vi "运维调试_氨氮.vi"() -> ()   [LabVIEW 2016, in "斯坦道氨氮.lvlib"]
uses:
  <vilib>/Utility/miscctls.llb/LVPointTypeDef.ctl
  <vilib>/Utility/config.llb/NI_LVConfig.lvlib
  <vilib>/ptbypt/NI_PtbyPt.lvlib
panel:
  in  "仪器参数设置":bool
  in  "模块启用":bool
  in  "串口设置":bool
  in  "备用系数一键写入":bool
  in  "公式一键写入":bool
  in  "流程路径":path=path "C:/Users/STD/Documents/斯坦道流程文件/流程.xml"
  in  "曲线模型":cluster{"X^2":dbl, "X":dbl, "B":dbl}(xcontrol)
  out "字符串":string
  in  "质控参数设置":bool
  in  "自动测试量程配置":T1
  out "温度2":sgl
  out "温度1":sgl
  out "ADC":sgl
  out "固件版本号":string
  in  "数组":string[](array[string])
  in  "备用系数写入":bool
  in  "备用系数读取":bool
  in  "备用系数":T2
  in  "量程切换阈值写入":bool
  in  "量程切换阈值读取":bool
  in  "量程切换阈值":cluster{"阈值":dbl, "标液浓度":dbl}
  in  "参数下拉列表":enum16{"总磷", "总氮", "氨氮"}(ring)=enum."氨氮"
  in  "量程下拉列表":enum16{"低量程", "高量程"}(ring)
  in  "测量模式下拉列表":enum16{"水样测量", "零点核查", "跨度核查", "标样核查", "加标回收"}(ring)
  in  "公式":cluster{"X^2":dbl, "X":dbl, "b":dbl}
  in  "写公式":bool
  in  "读公式":bool
  in  "返回":bool
  in  "设置":bool
  out "序列号":string="序列号"
  out "测量数据":T3(xcontrol)
  out "集成报警信息":string
  out "定时启动":bool
  out "运行状态":T4(xcontrol)
  in  "停止":bool
  in  "手动启动":bool
  in  "单步测试":bool
  in  "总磷氨氮调试":u16[](xcontrol)
  out "F3":sgl format="%#.6f"
  out "F2":sgl format="%#.6f"
  out "F1":sgl format="%#.6f"
  out "F0":sgl format="%#.6f"
  out "多列列表框":i32(listbox)
  # "参数设置"
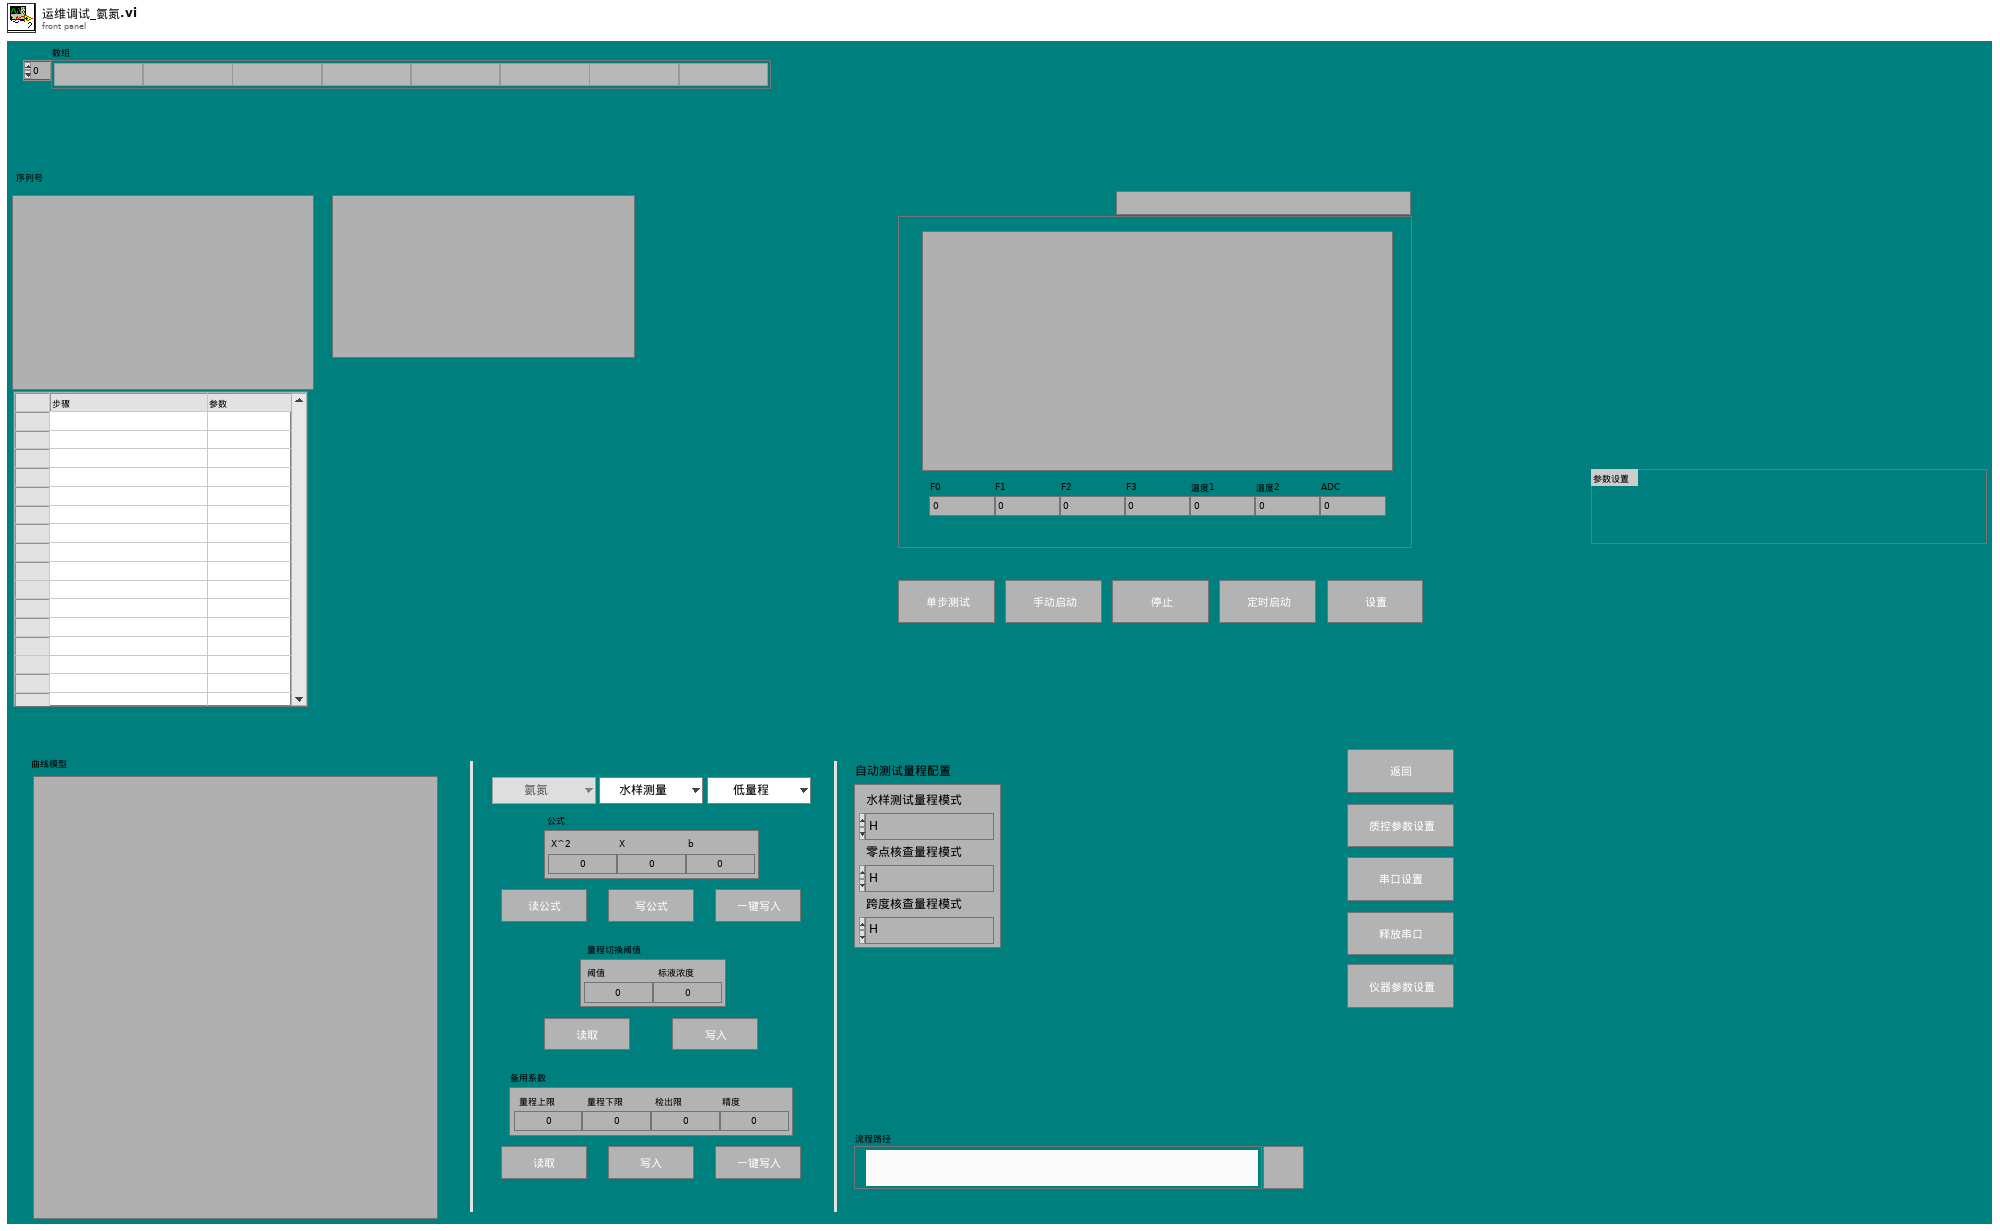
[diagram p1: front panel]
types:
  T1 = cluster{"水样测试量程模式":enum16{"H", "L", "AUTO"}, "空白核查量程模式":enum16{"H", "L", "AUTO"}, "跨度核查量程模式":enum16{"H", "L", "AUTO"}}
  T2 = cluster{"量程上限":dbl, "量程下限":dbl, "检出限":dbl, "精度":dbl}
  T3 = cluster{"flowid":u16, "测量精度":u16, "测量数据区":cluster{"因子编码":u32, "单位":u16, "标样参考值":sgl, "水样数据时间":timestamp, "水样实测值":sgl, "水样数据标识":string, "标样数据时间":timestamp, "标样实测值":sgl, "标样数据标识":string, "空白数据时间":timestamp, "空白实测值":sgl, "空白数据标识":string, "零点核查数据时间":timestamp, "零点核查实测值":sgl, "零点核查数据标识":string, "跨度核查数据时间":timestamp, "跨度核查实测值":sgl, "跨度核查数据标识":string, "加标回收数据时间":timestamp, "加标回收实测值":sgl, "加标回收数据标识":string, "平行样数据时间":timestamp, "平行样实测值":sgl, "平行样数据标识":string, "F0":sgl, "F1":sgl, "F2":sgl, "F3":sgl, "F4":sgl, "F5":sgl, "F6":sgl, "F7":sgl, "温度":sgl, "湿度":sgl, "X值":sgl}}
  T4 = cluster{"系统时间":timestamp, "工作状态":enum16{"空闲", "水样测试", "标样核查", "零点核查", "跨度核查", "空白测试", "平行样测试", "加标回收", "空白校准", "标样校准", "初始化（清洗）"}, "测量模式":enum16{"待机", "连续模式", "周期模式", "定点模式", "受控模式", "手动模式"}, "告警代码":enum16{"无告警", "缺试剂告警", "缺水样告警", "缺蒸馏水告警", "缺标液告警", "仪表漏液告警", "标定异常告警", "超量程告警", "加热异常", "低试剂预警", "超上限告警", "超下限告警", "仪表内部其他异常", "滴定异常告警", "电极异常告警", "量程切换告警", "参数设置告警", "PH电极电位异常", "电导率电极异常", "浊度光度异常", "溶解氧电极异常", "溶解氧光强异常", "温度异常告警", "PH异常告警", "溶解氧异常告警", "电导率异常告警", "浊度异常告警", "叶绿素异常告警", "藻密度异常告警", "蓝绿藻异常告警", "ORP异常告警", "氨氮异常告警", "清洁刷异常告警", "SD卡异常告警", "蓝牙异常告警", "Wifi异常告警", "流程异常告警"}, "故障代码":enum16{"无故障", "电机故障", "温度故障", "通讯故障", "滴定故障"}, "日志代码":u16, "软件版本":u16, "F0":sgl, "F1":sgl, "F2":sgl, "F3":sgl, "T":sgl, "H":sgl, "id":u16, "flowid":u16, "量程":u16, "总磷控温温度1":sgl, "营养盐控温温度2":sgl, "ADC":sgl}
  T5 = enum16{"启动测量", "标样核查", "零点核查", "跨度核查", "空白测试", "平行样测试", "加标回收", "空白校准", "标样校准", "初始化（清洗）", "停止测试", "仪器重启", "校时", "模式设置", "测量间隔设置"}
  T6 = cluster{"控制命令":enum16{"启动测量", "标样核查", "零点核查", "跨度核查", "空白测试", "平行样测试", "加标回收", "空白校准", "标样校准", "初始化（清洗）", "停止测试", "仪器重启", "校时", "模式设置", "测量间隔设置"}, "周期设置类型":enum16{"定点启动", "间隔启动"}, "定时功能启用":bool, "定时间隔":dbl, "24H周期设置":bool[], "零点核查时间":u16, "跨度核查时间":u16, "质控频次":enum16{"关闭", "每天", "星期一", "星期二", "星期三", "星期四", "星期五", "星期六", "星期日"}}
  T7 = enum16{"关闭", "每天", "星期一", "星期二", "星期三", "星期四", "星期五", "星期六", "星期日"}
  T8 = typedef "LVDateTimeRec.ctl" = cluster{"秒数的小数部分":dbl, "秒":i32, "分":i32, "时":i32, "日":i32, "月":i32, "年":i32, "天数（周）":i32, "天数（年）":i32, "DST":i32}
  T9 = enum16{"空闲", "水样测试", "标样核查", "零点核查", "跨度核查", "空白测试", "平行样测试", "加标回收", "空白校准", "标样校准", "初始化（清洗）"}
  T10 = enum32{"Bad", "Idle", "Run top level", "Running"}
  T11 = typedef "LVPointTypeDef.ctl" = cluster{"Horizontal":i16, "Vertical":i16}
  T12 = cluster{"因子编码":u32, "单位":u16, "标样参考值":sgl, "水样数据时间":timestamp, "水样实测值":sgl, "水样数据标识":string, "标样数据时间":timestamp, "标样实测值":sgl, "标样数据标识":string, "空白数据时间":timestamp, "空白实测值":sgl, "空白数据标识":string, "零点核查数据时间":timestamp, "零点核查实测值":sgl, "零点核查数据标识":string, "跨度核查数据时间":timestamp, "跨度核查实测值":sgl, "跨度核查数据标识":string, "加标回收数据时间":timestamp, "加标回收实测值":sgl, "加标回收数据标识":string, "平行样数据时间":timestamp, "平行样实测值":sgl, "平行样数据标识":string, "F0":sgl, "F1":sgl, "F2":sgl, "F3":sgl, "F4":sgl, "F5":sgl, "F6":sgl, "F7":sgl, "温度":sgl, "湿度":sgl, "X值":sgl}
  T13 = typedef "NI_LVConfig.lvlib/Config Data RefNum.ctl" = refnum<k1>
  T14 = cluster{"参数下拉列表":enum16{"总磷", "总氮", "氨氮"}, "测量模式下拉列表":enum16{"水样测量", "零点核查", "跨度核查", "标样核查", "加标回收"}, "量程下拉列表":enum16{"低量程", "高量程"}}
  T15 = cluster{"启动模式":enum16{"跨度核查", "水样测量", "空白核查", "标样核查", "加标回收"}, "启动参数":u16, "量程":enum16{"低量程", "高量程"}}
  T16 = cluster{"时间标识":timestamp, "设备":string, "日志信息":string, "流程参数":string}
  T17 = cluster{"时间标识":timestamp, "设备":string, "日志信息":string}
  T18 = enum16{"无告警", "缺试剂告警", "缺水样告警", "缺蒸馏水告警", "缺标液告警", "仪表漏液告警", "标定异常告警", "超量程告警", "加热异常", "低试剂预警", "超上限告警", "超下限告警", "仪表内部其他异常", "滴定异常告警", "电极异常告警", "量程切换告警", "参数设置告警", "PH电极电位异常", "电导率电极异常", "浊度光度异常", "溶解氧电极异常", "溶解氧光强异常", "温度异常告警", "PH异常告警", "溶解氧异常告警", "电导率异常告警", "浊度异常告警", "叶绿素异常告警", "藻密度异常告警", "蓝绿藻异常告警", "ORP异常告警", "氨氮异常告警", "清洁刷异常告警", "SD卡异常告警", "蓝牙异常告警", "Wifi异常告警", "流程异常告警"}
  T19 = typedef "LVRowAndColumnUnsignedTypeDef.ctl" = cluster{"Row":u32, "Column":u32}
  T20 = cluster{"站号":u16, "量程切换":enum32{"H", "L", "AUTO"}, "控制命令":enum16{"启动测量", "标样核查", "零点核查", "跨度核查", "空白测试", "平行样测试", "加标回收", "空白校准", "标样校准", "初始化（清洗）", "停止测试", "仪器重启", "校时", "模式设置", "测量间隔设置"}, "模式设置":enum16{"待机", "连续模式", "周期模式", "定点模式", "受控模式", "手动模式"}, "测量间隔":u16}
  T21 = cluster{"氨氮跨度值":dbl, "氨氮零点标准液浓度":dbl, "氨氮跨度标准液浓度":dbl, "氨氮标准液标准浓度":dbl}
  T22 = cluster{"确定":bool, "跨度值":dbl, "零点标准液浓度":dbl, "跨度标准液浓度":dbl, "标准液标准浓度":dbl}
  T23 = cluster{"测量量程":dbl, "测量精度":dbl, "测量间隔":dbl, "消解温度":dbl, "消解时长":dbl, "空白校准时间":timestamp, "曲线截距":dbl, "曲线斜率":dbl, "测量检出限":dbl, "测量信号值":dbl, "线性相关系数":dbl, "二次多项式系数":dbl, "标样校准时间":timestamp, "单位":u16}
  T24 = cluster{"确定":bool, "测量量程":dbl, "测量精度":dbl, "测量间隔":dbl, "消解温度":dbl, "消解时长":dbl, "空白校准时间":timestamp, "曲线截距":dbl, "曲线斜率":dbl, "测量检出限":dbl, "测量信号值":dbl, "线性相关系数":dbl, "二次多项式系数":dbl, "标样校准时间":timestamp, "单位":u16}
  T25 = cluster{"控制命令":enum16{"启动测量", "标样核查", "零点核查", "跨度核查", "空白测试", "平行样测试", "加标回收", "空白校准", "标样校准", "初始化（清洗）", "停止测试", "仪器重启", "校时", "模式设置", "测量间隔设置"}, "周期设置类型":enum16{"定点启动", "间隔启动"}, "定时功能启用":bool, "定时间隔":dbl, "24H周期设置":bool[], "空白核查时间":u16, "跨度核查时间":u16, "质控频次":enum16{"关闭", "每天", "星期一", "星期二", "星期三", "星期四", "星期五", "星期六", "星期日"}}
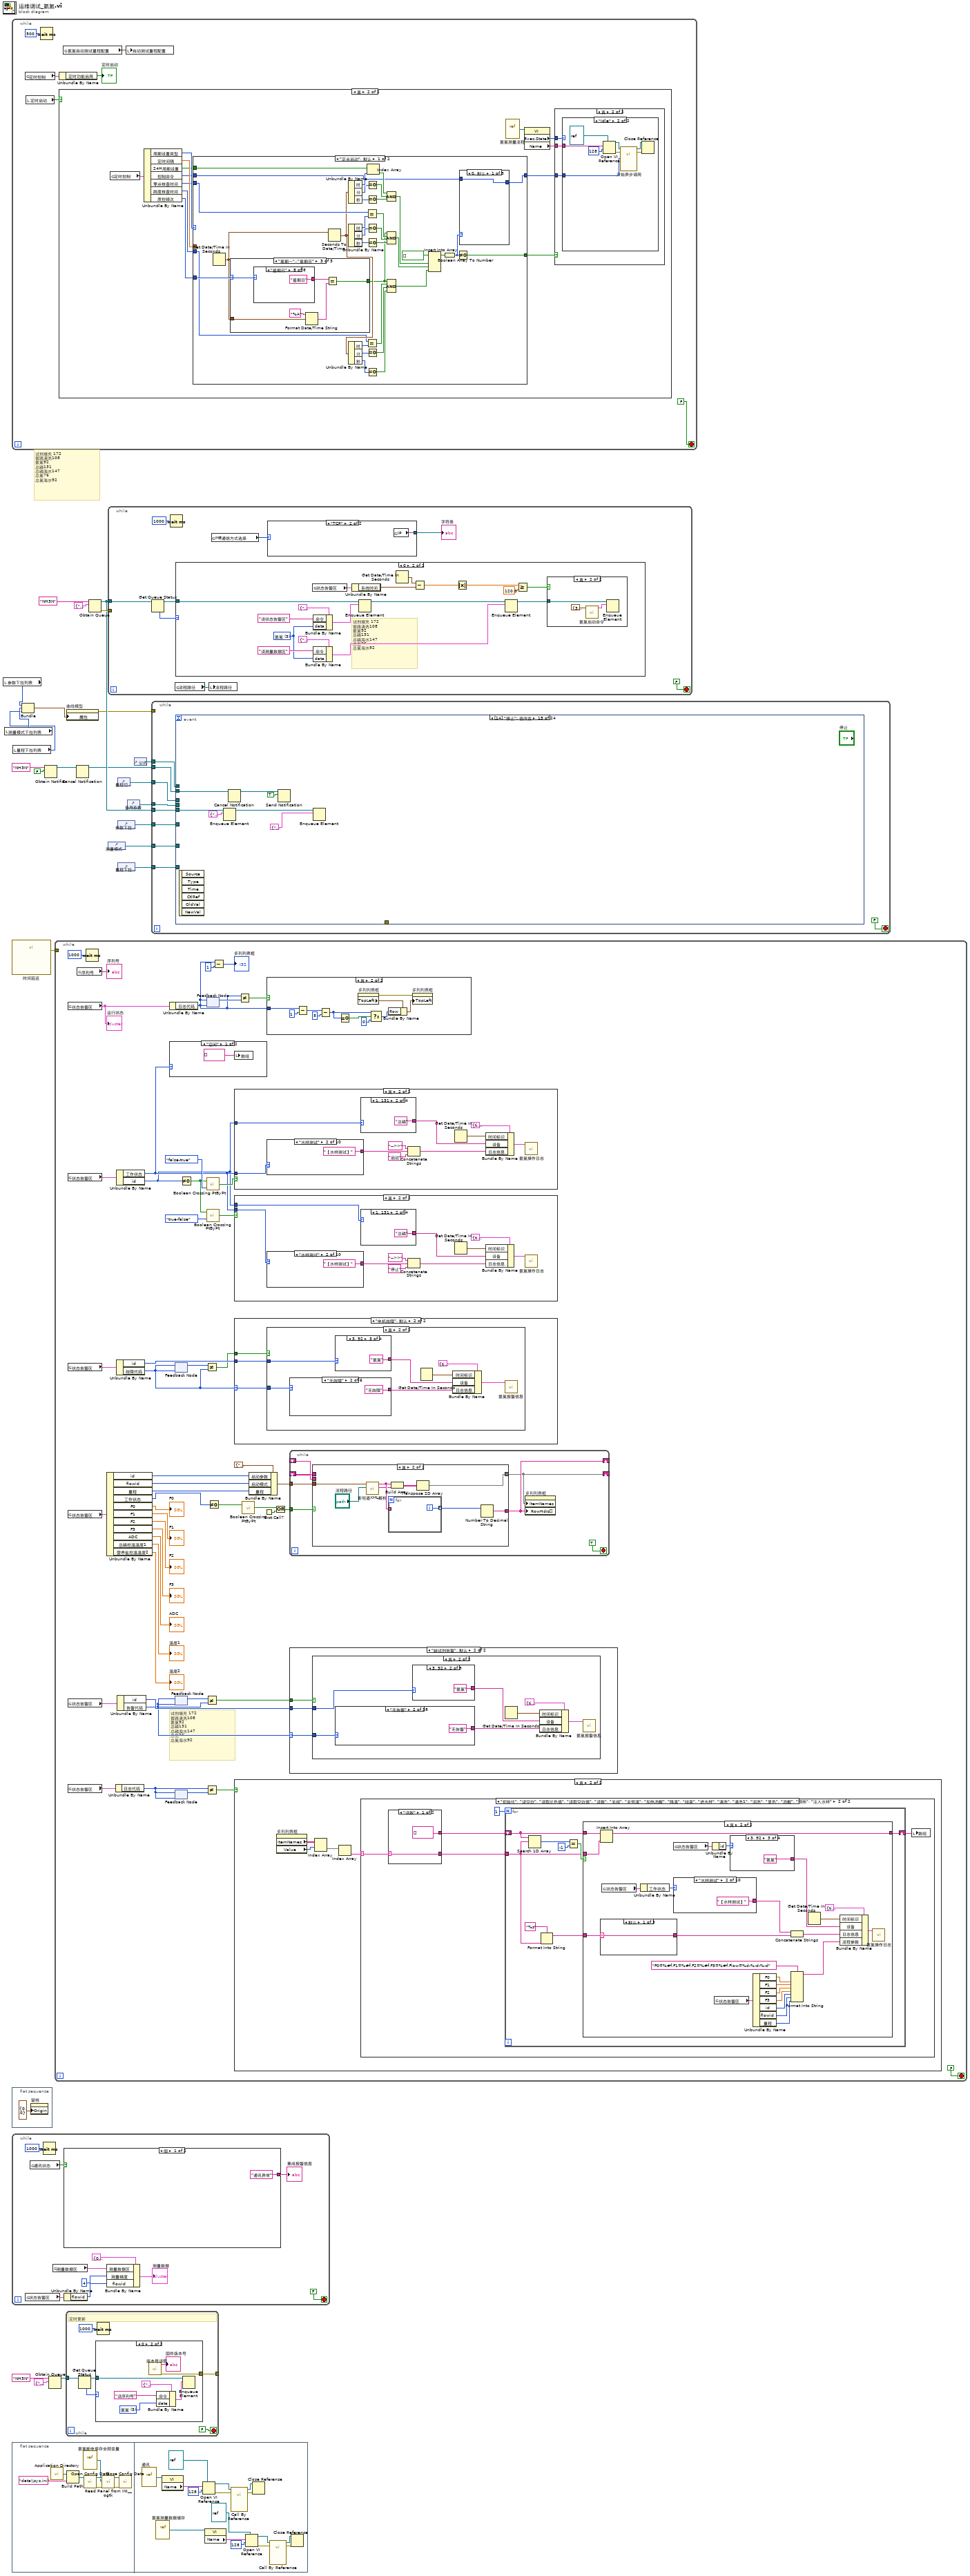
[diagram p0: block diagram]
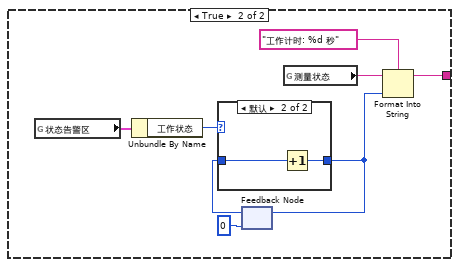
[diagram p3: hidden frame]
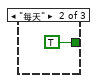
[diagram p9: hidden frame]
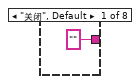
[diagram p10: hidden frame]
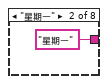
[diagram p11: hidden frame]
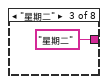
[diagram p12: hidden frame]
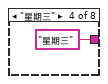
[diagram p13: hidden frame]
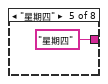
[diagram p14: hidden frame]
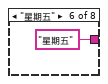
[diagram p15: hidden frame]
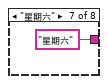
[diagram p16: hidden frame]
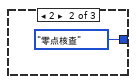
[diagram p17: hidden frame]
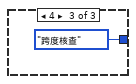
[diagram p18: hidden frame]
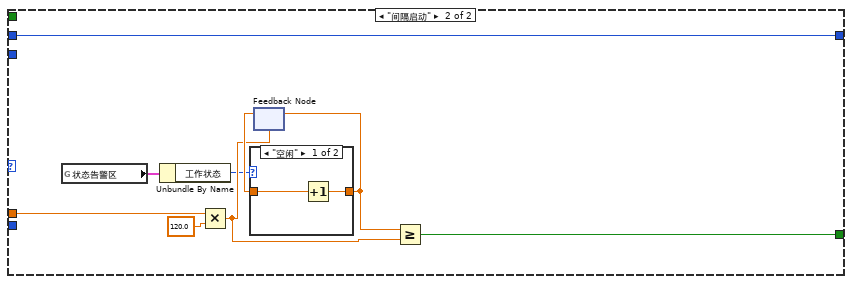
[diagram p19: hidden frame]
diagram:
  # "试剂填充 172 \n管路清洗108\n氨氮92\n总磷131\n总磷海水147\n总氮76\n总氮海水92"
  n1 = local read "参数下拉列表"() -> (w4:enum16{"总磷", "总氮", "氨氮"})
  n2 = local read "测量模式下拉列表"() -> (w3:enum16{"水样测量", "零点核查", "跨度核查", "标样核查", "加标回收"})
  n3 = while {
    stop <- FALSE stop-if-true
    n4 = global read "氨氮断电保存全局变量.vi" "定时控制"() -> (w25:T6)
    n5 = local read "定时启动"() -> (w27:bool)
    n6 = Wait (ms)(milliseconds to wait=u32 500 ("等待时间（毫秒）")) -> ()  [unwired: 1 out]
    n7 = Unbundle By Name(w25) -> ("定时功能启用"=→"定时启动":bool)
    n8 = case shown="真" w27 {
      frame False {
      }
      frame True {
        n9 = global read "氨氮断电保存全局变量.vi" "定时控制"() -> (w42:T6)
        n10 = Unbundle By Name(w42) -> ("周期设置类型"=w41:enum16{"定点启动", "间隔启动"}, "定时间隔"=w40:dbl, "24H周期设置"=w39:bool[], "控制命令"=w34:T5, "零点核查时间"=w32:u16, "跨度核查时间"=w31:u16, "质控频次"=w30:T7)
        n11 = case shown="\"定点启动\", 默认" w41 {
          tunnel: w40 -> [_ w112]
          tunnel: w39 -> [w78 _]
          tunnel: [w56 w110] -> w38
          tunnel: w34 -> [w54 w108]
          tunnel: [w82 w108] -> w33
          tunnel: w30 -> [w81 _]
          tunnel: w32 -> [w74 _]
          tunnel: w31 -> [w63 _]
          frame "定点启动", Default {
            n12 = Get Date/Time In Seconds() -> (seconds since 1Jan1904=w80:timestamp)
            n13 = case shown="\"星期一\"..\"星期日\"" w81 {
              selector: w81 -> [_ _ w92]
              tunnel: w80 -> [_ _ w93]
              tunnel: [_ TRUE w89] -> w62
              frame "关闭", Default {
              }
              frame "每天" {
              }
              frame "星期一".."星期日" {
                n14 = case shown="\"星期日\"" w92 {
                  tunnel: ["" ("时间格式字符串(%c)") "星期一" ("时间格式字符串(%c)") "星期二" ("时间格式字符串(%c)") "星期三" ("时间格式字符串(%c)") "星期四" ("时间格式字符串(%c)") "星期五" ("时间格式字符串(%c)") "星期六" ("时间格式字符串(%c)") "星期日" ("时间格式字符串(%c)")] -> w91
                  frame "关闭", Default {
                  }
                  frame "星期一" {
                  }
                  frame "星期二" {
                  }
                  frame "星期三" {
                  }
                  frame "星期四" {
                  }
                  frame "星期五" {
                  }
                  frame "星期六" {
                  }
                  frame "星期日" {
                  }
                }
                n15 = Format Date/Time String(time format string (%c)="%A" ("时间格式字符串(%c)"), seconds (now)=w93) -> (date/time string=w90:string)  [unwired: 1 in]
                n16 = Equal?(x=w91, y=w90) -> (x = y?=w89:bool)
              }
            }
            n17 = Seconds To Date/Time(time stamp (now)=w80) -> (date time rec=w64:T8)  [unwired: 1 in]
            n18 = Unbundle By Name(w64) -> ("时"=w87:i32, "分"=w85:i32, "秒"=w86:i32)
            n19 = Unbundle By Name(w64) -> ("时"=w75:i32, "分"=w77:i32, "秒"=w76:i32)
            n20 = Unbundle By Name(w64) -> ("时"=w67:i32, "分"=w65:i32, "秒"=w66:i32)
            n21 = Equal?(x=w74, y=w75) -> (x = y?=w73:bool)
            n22 = Equal?(x=w63, y=w67) -> (x = y?=w68:bool)
            n23 = Equal To 0?(x=w85) -> (x = 0?=w84:bool)
            n24 = Equal To 0?(x=w86) -> (x = 0?=w83:bool)
            n25 = Equal To 0?(x=w77) -> (x = 0?=w72:bool)
            n26 = Equal To 0?(x=w76) -> (x = 0?=w71:bool)
            n27 = Equal To 0?(x=w65) -> (x = 0?=w69:bool)
            n28 = Equal To 0?(x=w66) -> (x = 0?=w70:bool)
            n29 = Index Array(array=w78, index=w87) -> (element=w79:bool)
            n30 = Compound Arithmetic op=AND ("复合运算")(w79, w84, w83) -> (w60:bool)
            n31 = Compound Arithmetic op=AND ("复合运算")(w62, w73, w72, w71) -> (w59:bool)
            n32 = Compound Arithmetic op=AND ("复合运算")(w62, w68, w69, w70) -> (w58:bool)
            n33 = Insert Into Array(array=bool[] [], new element #1=w60, new element #2=w59, new element #3=w58) -> (w57:bool[])  [unwired: 1 in]
            n34 = Boolean Array To Number(Boolean array=w57) -> (number=w55:u32)
            n35 = Not Equal To 0?(x=w55) -> (x != 0?=w56:bool)
            n36 = case shown="0, 默认" w55 {
              tunnel: [w103 T5."零点核查" ("控制命令") T5."跨度核查" ("控制命令")] -> w82
              tunnel: w54 -> [w103 _ _]
              frame 0, Default {
              }
              frame 2 {
              }
              frame 4 {
              }
            }
          }
          frame "间隔启动" {
            n37 = global read "VAR氨氮全局变量.vi" "状态告警区"() -> (w107:T4)
            n38 = Unbundle By Name(w107) -> ("工作状态"=w106:T9)
            n39 = Multiply(x=w112, y=120.0) -> (x*y=w109:dbl)
            n40 = feedback #1(w109) -> (w114:dbl)
            n41 = case shown="\"空闲\"" w106 {
              tunnel: w114 -> [w116 _]
              tunnel: [w115 _] -> w113
              frame "空闲" {
                n42 = Increment(x=w116) -> (x+1=w115:dbl)
              }
              frame "水样测试", Default {
              }
            }
            n43 = feedback-in #1(w113) -> ()
            n44 = Greater Or Equal?(x=w113, y=w109) -> (x >= y?=w110:bool)
          }
        }
        n45 = vi-ref "氨氮测量流程.vi"() -> (w37:refnum<vi>)
        n46 = property class="VI"(reference=w37) -> ("Exec.State"=w36:T10, "Name"=w35:string)  [unwired: 1 in, 2 out]
        n47 = case shown="真" w38 {
          tunnel: w35 -> [_ w45]
          tunnel: w33 -> [_ w44]
          tunnel: w36 -> [_ w43]
          frame False {
          }
          frame True {
            n48 = case shown="\"Idle\"" w43 {
              tunnel: w45 -> [_ w49]
              tunnel: w44 -> [_ w47]
              frame "Bad", Default {
              }
              frame "Idle" {
                n49 = Open VI Reference(type specifier VI Refnum (for type only)=refnum<vi> refnum, vi path=w49, options=128 ("选项")) -> (vi reference=w50:refnum<vi>, error out=w51:errorcluster)  [unwired: 3 in]
                n50 = call-by-ref "开始异步调用"(reference=w50, error in=w51, "控制命令"=w47) -> (reference out=w52:refnum<vi>, error out=w53:errorcluster)  [unwired: 11 in]
                n51 = Close Reference(reference=w52, error in (no error)=w53) -> ()  [unwired: 1 out]
              }
            }
          }
        }
      }
    }
    n52 = global read "氨氮断电保存全局变量.vi" "氨氮自动测试量程配置"() -> (w26:T1)
    n53 = local write "自动测试量程配置"(w26) -> ()
  }
  n54 = call "时间延迟"() -> ("error out"=w13:errorcluster)  [unwired: 11 in]
  n55 = flat-sequence {
    frame #0 {
      n56 = property on="窗格" class="Pane"("Origin"=T11 {"Horizontal"=0, "Vertical"=0} ("原点")) -> ()  [unwired: 2 in, 2 out]
    }
  }
  n57 = while {
    stop <- FALSE stop-if-true
    n58 = global read "VAR氨氮全局变量.vi" "状态告警区"() -> (w123:T4)
    n59 = global read "VAR氨氮全局变量.vi" "通讯状态"() -> (w125:bool)
    n60 = Wait (ms)(milliseconds to wait=u32 1000 ("等待时间（毫秒）")) -> ()  [unwired: 1 out]
    n61 = global read "VAR氨氮全局变量.vi" "测量数据区"() -> (w118:T12)
    n62 = case shown="假" w125 {
      tunnel: ["通讯异常" ("集成报警信息") w130] -> w124
      frame False {
      }
      frame True {
        n63 = global read "VAR氨氮全局变量.vi" "状态告警区"() -> (w136:T4)
        n64 = Unbundle By Name(w136) -> ("工作状态"=w135:T9)
        n65 = feedback #2(0) -> (w133:i32)
        n66 = case shown="默认" w135 {
          tunnel: w133 -> [_ w138]
          tunnel: [_ w137] -> w131
          frame "空闲" {
          }
          frame Default {
            n67 = Increment(x=w138) -> (x+1=w137:i32)
          }
        }
        n68 = feedback-in #2(w131) -> ()
        n69 = global read "VAR氨氮全局变量.vi" "测量状态"() -> (w129:string)
        n70 = Format Into String(format string="工作计时: %d 秒" ("格式字符串"), initial string=w129, w131) -> (resulting string=w130:string)  [unwired: 1 in, 1 out]
      }
    }
    "集成报警信息" <- w124
    n71 = Unbundle By Name(w123) -> ("flowid"=w122:u16)
    n72 = Bundle By Name(cluster=T3 {"flowid"=0, "测量精度"=0, "测量数据区"={"因子编码"=0, "单位"=0, "标样参考值"=0.0, "水样数据时间"=timestamp(0 s since 1904-01-01), "水样实测值"=0.0, "水样数据标识"="", "标样数据时间"=timestamp(0 s since 1904-01-01), "标样实测值"=0.0, "标样数据标识"="", "空白数据时间"=timestamp(0 s since 1904-01-01), "空白实测值"=0.0, "空白数据标识"="", "零点核查数据时间"=timestamp(0 s since 1904-01-01), "零点核查实测值"=0.0, "零点核查数据标识"="", "跨度核查数据时间"=timestamp(0 s since 1904-01-01), "跨度核查实测值"=0.0, "跨度核查数据标识"="", "加标回收数据时间"=timestamp(0 s since 1904-01-01), "加标回收实测值"=0.0, "加标回收数据标识"="", "平行样数据时间"=timestamp(0 s since 1904-01-01), "平行样实测值"=0.0, "平行样数据标识"="", "F0"=0.0, "F1"=0.0, "F2"=0.0, "F3"=0.0, "F4"=0.0, "F5"=0.0, "F6"=0.0, "F7"=0.0, "温度"=0.0, "湿度"=0.0, "X值"=0.0}} ("总氮测量数据"), "测量数据区"=w118, "测量精度"=u16 4, "flowid"=w122) -> (→"测量数据":T3)
  }
  n73 = flat-sequence {
    frame #0 {
      n74 = call <vilib>:"Application Directory.vi"() -> ("Application Directory"=w146:path)
      n75 = Build Path(base path=w146, name or relative path="data\\sys.ini" ("名称或相对路径")) -> (appended path=w144:path)
      n76 = vi-ref "氨氮断电保存全局变量.vi"() -> (w142:refnum<vi>)
      n77 = call <vilib>:"Open Config Data.vi"("configuration file path"=w144) -> ("error out"=w140:errorcluster, "refnum"=w143:T13)  [unwired: 8 in, 1 out]
      n78 = call <userlib>:"Read Panel from INI__ogtk.vi"("error in (no error)"=w140, "VI ref"=w142, "refnum"=w143) -> ("error out"=w139:errorcluster, "refnum out"=w141:T13)  [unwired: 7 in]
      n79 = call <vilib>:"Close Config Data.vi"("error in (no error)"=w139, "refnum"=w141) -> ()  [unwired: 8 in, 2 out]
    }
    frame #1 {
      n80 = vi-ref "通讯.vi"() -> (w162:refnum<vi>)
      n81 = vi-ref "氨氮测量数据储存.vi"() -> (w154:refnum<vi>)
      n82 = property class="VI"(reference=w162) -> ("Name"=w161:string)  [unwired: 1 in, 2 out]
      n83 = Open VI Reference(type specifier VI Refnum (for type only)=refnum<vi> refnum, vi path=w161, options=128 ("选项")) -> (vi reference=w159:refnum<vi>, error out=w157:errorcluster)  [unwired: 3 in]
      n84 = property class="VI"(reference=w154) -> ("Name"=w147:string)  [unwired: 1 in, 2 out]
      n85 = call-by-ref "?"(reference=w159, error in=w157) -> (reference out=w155:refnum<vi>, error out=w156:errorcluster)  [unwired: 12 in]
      n86 = Open VI Reference(type specifier VI Refnum (for type only)=refnum<vi> refnum, vi path=w147, options=128 ("选项")) -> (vi reference=w149:refnum<vi>, error out=w151:errorcluster)  [unwired: 3 in]
      n87 = Close Reference(reference=w155, error in (no error)=w156) -> ()  [unwired: 1 out]
      n88 = call-by-ref "?"(reference=w149, error in=w151) -> (reference out=w153:refnum<vi>, error out=w152:errorcluster)  [unwired: 12 in]
      n89 = Close Reference(reference=w153, error in (no error)=w152) -> ()  [unwired: 1 out]
    }
  }
  n90 = local read "量程下拉列表"() -> (w2:enum16{"低量程", "高量程"})
  n91 = Bundle("参数下拉列表"=w4, "测量模式下拉列表"=w3, "量程下拉列表"=w2) -> (w1:T14)  [unwired: 1 in]
  n92 = Obtain Notifier(name (unnamed)="NH3N" ("名称（未命名）"), notification data type=FALSE) -> (notifier out=w6:refnum<notifier>)  [unwired: 2 in, 2 out]
  n93 = Obtain Queue(name (unnamed)="NH3N" ("名称（未命名）"), element data type=cluster{"命令":string, "data":variant} {"命令"="", "data"=variant}) -> (queue out=w10:refnum<queue>)  [unwired: 3 in, 2 out]
  n94 = while {
    tunnel: w13 -> [_]
    stop <- FALSE stop-if-true
    # "试剂填充 172 \n管路清洗108\n氨氮92\n总磷131\n总磷海水147\n总氮76\n总氮海水92"
    n95 = global read "VAR氨氮全局变量.vi" "状态告警区"() -> (w196:T4)
    "运行状态" <- w196
    n96 = global read "VAR氨氮全局变量.vi" "状态告警区"() -> (w183:T4)
    n97 = global read "VAR氨氮全局变量.vi" "状态告警区"() -> (w188:T4)
    n98 = global read "VAR氨氮全局变量.vi" "状态告警区"() -> (w204:T4)
    n99 = global read "VAR氨氮全局变量.vi" "状态告警区"() -> (w193:T4)
    n100 = global read "VAR氨氮全局变量.vi" "状态告警区"() -> (w181:T4)
    n101 = global read "VAR氨氮全局变量.vi" "序列号"() -> (→"序列号":string)
    n102 = Wait (ms)(milliseconds to wait=u32 1000 ("等待时间（毫秒）")) -> ()  [unwired: 1 out]
    n103 = Unbundle By Name(w204) -> ("id"=w201:u16, "flowid"=w203:u16, "量程"=w202:u16, "工作状态"=w171:T9, "F0"=→"F0":sgl, "F1"=→"F1":sgl, "F2"=→"F2":sgl, "F3"=→"F3":sgl, "ADC"=→"ADC":sgl, "总磷控温温度1"=→"温度1":sgl, "营养盐控温温度2"=→"温度2":sgl)
    n104 = Unbundle By Name(w181) -> ("日志代码"=w180:u16)
    n105 = Unbundle By Name(w183) -> ("工作状态"=w167:T9, "id"=w166:u16)
    n106 = Unbundle By Name(w188) -> ("id"=w187:u16, "故障代码"=w184:enum16{"无故障", "电机故障", "温度故障", "通讯故障", "滴定故障"})
    n107 = Unbundle By Name(w193) -> ("id"=w192:u16, "告警代码"=w189:T18)
    n108 = Unbundle By Name(w196) -> ("日志代码"=w177:u16)
    n109 = case shown="\"空闲\"" w167 {
      frame "空闲" {
        n110 = local write "数组"(string[] [] ("数组")) -> ()
      }
      frame "水样测试", Default {
      }
    }
    n111 = feedback #3(w184) -> (w185:enum16{"无故障", "电机故障", "温度故障", "通讯故障", "滴定故障"})
    n112 = feedback-in #3(w184) -> ()
    n113 = feedback #4(w189) -> (w190:T18)
    n114 = feedback-in #4(w189) -> ()
    n115 = feedback #5(w180) -> (w182:u16)
    n116 = feedback-in #5(w180) -> ()
    n117 = Not Equal To 0?(x=w166) -> (x != 0?=w164:bool)
    n118 = Not Equal?(x=w185, y=w184) -> (x != y?=w186:bool)
    n119 = Not Equal?(x=w190, y=w189) -> (x != y?=w191:bool)
    n120 = Not Equal?(x=w180, y=w182) -> (x != y?=w179:bool)
    n121 = feedback-in #6(w177) -> ()
    n122 = feedback #6(w177) -> (w209:u16)
    n123 = call <vilib>:"Boolean Crossing PtByPt.vi"("direction"=enum16{"either", "false-true", "true-false"}."false-true", "input"=w164) -> ("crossing"=w168:bool)  [unwired: 1 in]
    n124 = call <vilib>:"Boolean Crossing PtByPt.vi"("direction"=enum16{"either", "false-true", "true-false"}."true-false", "input"=w164) -> ("crossing"=w163:bool)  [unwired: 1 in]
    n125 = Not Equal To 0?(x=w171) -> (x != 0?=w206:bool)
    n126 = Subtract(x=w177, y=1) -> (x-y=→"多列列表框":i32)
    n127 = case shown="真" w168 {
      tunnel: w166 -> [_ w236]
      tunnel: w167 -> [_ w235]
      frame False {
      }
      frame True {
        n128 = case shown="\"水样测试\"" w235 {
          tunnel: [_ "【水样测试】" ("字符串") "【标样核查】" ("字符串") "【零点核查】" ("字符串") "【跨度核查】" ("字符串") "【空白测试】" ("字符串") "【平行样测试】" ("字符串") "【加标回收】" ("字符串") "【空白校准】" ("字符串") "【标样校准】" ("字符串")] -> w240
          frame "空闲", Default {
          }
          frame "水样测试" {
          }
          frame "标样核查" {
          }
          frame "零点核查" {
          }
          frame "跨度核查" {
          }
          frame "空白测试" {
          }
          frame "平行样测试" {
          }
          frame "加标回收" {
          }
          frame "空白校准" {
          }
          frame "标样校准" {
          }
        }
        n129 = case shown="1, 131" w236 {
          tunnel: [_ "总磷" ("table输入") "氨氮" ("table输入") "总氮" ("table输入")] -> w241
          frame Default {
          }
          frame 1, 131 {
          }
          frame 3, 92 {
          }
          frame 2, 76 {
          }
        }
        n130 = Concatenate Strings("-->>" ("字符串"), w240, "启动" ("字符串")) -> (w239:string)
        n131 = Get Date/Time In Seconds() -> (seconds since 1Jan1904=w242:timestamp)
        n132 = Bundle By Name(cluster=T16 {"时间标识"=timestamp(0 s since 1904-01-01), "设备"="", "日志信息"="", "流程参数"=""} ("data in"), "时间标识"=w242, "设备"=w241, "日志信息"=w239) -> (w234:T16)
        n133 = call "氨氮操作日志.vi"("data in"=w234) -> ()  [unwired: 11 in]
      }
    }
    n134 = case shown="真" w163 {
      tunnel: w166 -> [_ w214]
      tunnel: w167 -> [_ w213]
      frame False {
      }
      frame True {
        n135 = case shown="\"水样测试\"" w213 {
          tunnel: [_ "【水样测试】" ("字符串") "【标样核查】" ("字符串") "【零点核查】" ("字符串") "【跨度核查】" ("字符串") "【空白测试】" ("字符串") "【平行样测试】" ("字符串") "【加标回收】" ("字符串") "【空白校准】" ("字符串") "【标样校准】" ("字符串")] -> w218
          frame "空闲", Default {
          }
          frame "水样测试" {
          }
          frame "标样核查" {
          }
          frame "零点核查" {
          }
          frame "跨度核查" {
          }
          frame "空白测试" {
          }
          frame "平行样测试" {
          }
          frame "加标回收" {
          }
          frame "空白校准" {
          }
          frame "标样校准" {
          }
        }
        n136 = case shown="1, 131" w214 {
          tunnel: [_ "总磷" ("table输入") "氨氮" ("table输入") "总氮" ("table输入")] -> w219
          frame Default {
          }
          frame 1, 131 {
          }
          frame 3, 92 {
          }
          frame 2, 76 {
          }
        }
        n137 = Concatenate Strings("-->>" ("字符串"), w218, "停止" ("字符串")) -> (w217:string)
        n138 = Get Date/Time In Seconds() -> (seconds since 1Jan1904=w220:timestamp)
        n139 = Bundle By Name(cluster=T16 {"时间标识"=timestamp(0 s since 1904-01-01), "设备"="", "日志信息"="", "流程参数"=""} ("data in"), "时间标识"=w220, "设备"=w219, "日志信息"=w217) -> (w212:T16)
        n140 = call "氨氮操作日志.vi"("data in"=w212) -> ()  [unwired: 11 in]
      }
    }
    n141 = case shown="\"电机故障\", 默认" w184 {
      selector: w184 -> [_ w324]
      tunnel: w187 -> [_ w325]
      tunnel: w186 -> [_ w323]
      frame "无故障" {
      }
      frame "电机故障", Default {
        n142 = case shown="真" w323 {
          tunnel: w325 -> [_ w332]
          tunnel: w324 -> [_ w327]
          frame False {
          }
          frame True {
            n143 = case shown="\"无故障\"" w327 {
              selector: w327 -> [w334 _ _ _ _ _]
              tunnel: [w333 "无故障" "电机故障" "温度故障" "通讯故障" "滴定故障"] -> w326
              frame Default {
                n144 = Format Into String(format string="%d" ("格式字符串"), initial string="未知" ("工作状态"), w334) -> (resulting string=w333:string)  [unwired: 1 in, 1 out]
              }
              frame "无故障" {
              }
              frame "电机故障" {
              }
              frame "温度故障" {
              }
              frame "通讯故障" {
              }
              frame "滴定故障" {
              }
            }
            n145 = case shown="3, 92" w332 {
              tunnel: [_ "总磷" ("table输入") "氨氮" ("table输入") "总氮" ("table输入")] -> w328
              frame Default {
              }
              frame 1, 131 {
              }
              frame 3, 92 {
              }
              frame 2, 76 {
              }
            }
            n146 = Get Date/Time In Seconds() -> (seconds since 1Jan1904=w329:timestamp)
            n147 = Bundle By Name(cluster=T17 {"时间标识"=timestamp(0 s since 1904-01-01), "设备"="", "日志信息"=""} ("data in"), "时间标识"=w329, "设备"=w328, "日志信息"=w326) -> (w330:T17)
            n148 = call "氨氮报警信息.vi"("data in"=w330) -> ()  [unwired: 10 in, 1 out]
          }
        }
      }
    }
    n149 = case shown="真" w179 {
      frame False {
      }
      frame True {
        n150 = property on="多列列表框" class="MCListbox (严格)"() -> ("ItemNames"=w259:string[][], "Value"=w260:i32)  [unwired: 2 in, 2 out]
        n151 = Index Array(array=w259, index (row)=w260) -> (element=w258:string[])  [unwired: 1 in]
        n152 = Index Array(array=w258) -> (element=w257:string)  [unwired: 1 in]
        n153 = case shown="\"初始化\", \"读空白\", \"读取比色值\", \"读取空白值\", \"读数\", \"关阀\", \"关恒温\", \"加热消解\", \"降温\", \"结束\", \"进水样\", \"清洗\", \"清洗1\", \"润洗\", \"显色\", \"消解\", \"预热\", \"注入水样\"" w257 {
          selector: w257 -> [_ w263]
          frame Default {
          }
          frame "初始化", "读空白", "读取比色值", "读取空白值", "读数", "关阀", "关恒温", "加热消解", "降温", "结束", "进水样", "清洗", "清洗1", "润洗", "显色", "消解", "预热", "注入水样" {
            n154 = case shown="\"读数\"" w263 {
              selector: w263 -> [w267 w269]
              tunnel: [w267 w269] -> w262
              tunnel: [string[] [] ("数组") "数组"] -> w261
              frame "读数" {
              }
              frame Default {
              }
            }
            n155 = for {
              N: 1 -> [_]
              tunnel: w262 -> [w271]
              shift-right: [w270] -> w264
              shift-left: w261 -> [w272]
              n156 = Search 1D Array(1D array=w272, element=w271) -> (index of element=w275:i32)  [unwired: 1 in]
              n157 = Format Into String(format string="%s" ("格式字符串"), w271) -> (resulting string=w276:string)  [unwired: 2 in, 1 out]
              n158 = Equal?(x=w275, y=-1) -> (x = y?=w273:bool)
              n159 = case shown="真" w273 {
                tunnel: w276 -> [_ w284]
                tunnel: w272 -> [w278 w288]
                tunnel: w271 -> [_ w287]
                tunnel: [w278 w286] -> w270
                frame False {
                }
                frame True {
                  n160 = Insert Into Array(array=w288, new element=w287) -> (w286:string[])  [unwired: 1 in]
                  n161 = case shown="默认" w284 {
                    selector: w284 -> [w313 w316 w319]
                    tunnel: [w313 w315 w318] -> w283
                    frame Default {
                    }
                    frame "初始化" {
                      n162 = Concatenate Strings("-->>" ("字符串"), w316) -> (w315:string)
                    }
                    frame "结束" {
                      n163 = Concatenate Strings("-->>" ("字符串"), w319) -> (w318:string)
                    }
                  }
                  n164 = global read "VAR氨氮全局变量.vi" "状态告警区"() -> (w282:T4)
                  n165 = Unbundle By Name(w282) -> ("工作状态"=w281:T9)
                  n166 = global read "VAR氨氮全局变量.vi" "状态告警区"() -> (w303:T4)
                  n167 = case shown="\"水样测试\"" w281 {
                    tunnel: [_ "【水样测试】" ("字符串") "【标样核查】" ("字符串") "【零点核查】" ("字符串") "【跨度核查】" ("字符串") "【空白测试】" ("字符串") "【平行样测试】" ("字符串") "【加标回收】" ("字符串") "【空白校准】" ("字符串") "【标样校准】" ("字符串")] -> w279
                    frame "空闲", Default {
                    }
                    frame "水样测试" {
                    }
                    frame "标样核查" {
                    }
                    frame "零点核查" {
                    }
                    frame "跨度核查" {
                    }
                    frame "空白测试" {
                    }
                    frame "平行样测试" {
                    }
                    frame "加标回收" {
                    }
                    frame "空白校准" {
                    }
                    frame "标样校准" {
                    }
                  }
                  n168 = Unbundle By Name(w303) -> ("id"=w302:u16)
                  n169 = global read "VAR氨氮全局变量.vi" "状态告警区"() -> (w298:T4)
                  n170 = case shown="3, 92" w302 {
                    tunnel: [_ "总磷" ("table输入") "氨氮" ("table输入") "总氮" ("table输入")] -> w300
                    frame Default {
                    }
                    frame 1, 131 {
                    }
                    frame 3, 92 {
                    }
                    frame 2, 76 {
                    }
                  }
                  n171 = Unbundle By Name(w298) -> ("F0"=w295:sgl, "F1"=w294:sgl, "F2"=w293:sgl, "F3"=w292:sgl, "id"=w291:u16, "flowid"=w290:u16, "量程"=w289:u16)
                  n172 = Concatenate Strings(w279, w283) -> (w280:string)
                  n173 = Format Into String(format string="F0=%#f,F1=%#f,F2=%#f,F3=%#f,Flow=%d-%-d-%-d" ("格式字符串"), w295, w294, w293, w292, w291, w290, w289) -> (resulting string=w296:string)  [unwired: 2 in, 1 out]
                  n174 = Get Date/Time In Seconds() -> (seconds since 1Jan1904=w299:timestamp)
                  n175 = Bundle By Name(cluster=T16 {"时间标识"=timestamp(0 s since 1904-01-01), "设备"="", "日志信息"="", "流程参数"=""} ("data in"), "时间标识"=w299, "设备"=w300, "日志信息"=w280, "流程参数"=w296) -> (w301:T16)
                  n176 = call "氨氮操作日志.vi"("data in"=w301) -> ()  [unwired: 11 in]
                }
              }
            }
            n177 = local write "数组"(w264) -> ()
          }
        }
      }
    }
    n178 = Not Equal?(x=w177, y=w209) -> (x != y?=w208:bool)
    n179 = call <vilib>:"Boolean Crossing PtByPt.vi"("input"=w206) -> ("crossing"=w170:bool)  [unwired: 2 in]
    n180 = Bundle By Name(cluster=T15 {"启动模式"=enum."跨度核查", "启动参数"=1, "量程"=enum."低量程"} ("参数簇"), "启动参数"=w201, "启动模式"=w203, "量程"=w202) -> (w195:T15)
    n181 = First Call?() -> (First Call?: T/F=w207:bool)
    n182 = case shown="真" w208 {
      tunnel: w177 -> [_ w419]
      frame False {
      }
      frame True {
        n183 = Subtract(x=w419, y=1) -> (x-y=w417:i32)
        n184 = Subtract(x=w417, y=5) -> (x-y=w421:i32)
        n185 = Greater Or Equal To 0?(x=w421) -> (x >= 0?=w420:bool)
        n186 = property on="多列列表框" class="MCListbox (严格)"() -> (error out=w425:errorcluster, "TopLeft"=w426:T19)  [unwired: 2 in, 1 out]
        n187 = Select(t=w421, s=w420, f=0) -> (s? t:f=w422:i32)
        n188 = Bundle By Name(cluster=w426, "Row"=w422) -> (w427:T19)
        n189 = property on="多列列表框" class="MCListbox (严格)"(error in=w425, "TopLeft"=w427) -> ()  [unwired: 1 in, 2 out]
      }
    }
    n190 = Or(x=w170, y=w207) -> (x .or. y?=w205:bool)
    n191 = while {
      tunnel: w205 -> [w405]
      tunnel: w195 -> [w404]
      shift-right: [w399] -> _
      shift-left: _ -> [w401]
      shift-right: [w400] -> _
      shift-left: _ -> [w402]
      stop <- TRUE stop-if-true
      n192 = case shown="真" w405 {
        tunnel: [w407 w415] -> w400
        tunnel: [w406 w414] -> w399
        tunnel: w404 -> [_ w409]
        tunnel: w402 -> [w407 _]
        tunnel: w401 -> [w406 _]
        frame False {
        }
        frame True {
          n193 = call "斯坦道XML解析.vi"("添加的路径"="流程路径", "参数簇"=w409) -> ("步骤时间"=w410:string[], "步骤名"=w412:string[])  [unwired: 8 in]
          n194 = for {
            tunnel: w412 -> [_] mode=indexing
            tunnel: [w416] -> w413 mode=indexing
            i -> [w416]
          }
          n195 = Build Array(w412, w410) -> (w411:string[][])
          n196 = Transpose 2D Array(2D array=w411) -> (transposed array=w414:string[][])
          n197 = Number To Decimal String(number=w413) -> (decimal integer string=w415:string[])  [unwired: 1 in]
        }
      }
      n198 = property on="多列列表框" class="MCListbox (严格)"("ItemNames"=w399, "RowHdrs[]"=w400) -> ()  [unwired: 2 in, 2 out]
    }
    n199 = case shown="\"缺试剂告警\", 默认" w189 {
      selector: w189 -> [_ w346]
      tunnel: w192 -> [_ w347]
      tunnel: w191 -> [_ w345]
      frame "无告警" {
      }
      frame "缺试剂告警", Default {
        n200 = case shown="真" w345 {
          tunnel: w347 -> [_ w354]
          tunnel: w346 -> [_ w348]
          frame False {
          }
          frame True {
            n201 = case shown="\"无告警\"" w348 {
              selector: w348 -> [w356 _ _ _ _ _ _ _ _ _ _ _ _ _ _ _ _ _ _ _ _ _ _ _ _ _ _ _ _ _ _ _ _ _ _ _ _ _]
              tunnel: [w355 "无告警" "缺试剂告警" "缺水样告警" "缺蒸馏水告警" "缺标液告警" "仪表漏液告警" "标定异常告警" "超量程告警" "加热异常" "低试剂预警" "超上限告警" "超下限告警" "仪表内部其他异常" "滴定异常告警" "电极异常告警" "量程切换告警" "参数设置告警" "PH电极电位异常" "电导率电极异常" "浊度光度异常" "溶解氧电极异常" "溶解氧光强异常" "温度异常告警" "PH异常告警" "溶解氧异常告警" "电导率异常告警" "浊度异常告警" "叶绿素异常告警" "藻密度异常告警" "蓝绿藻异常告警" "ORP异常告警" "氨氮异常告警" "清洁刷异常告警" "SD卡异常告警" "蓝牙异常告警" "WiFi异常告警" "流程异常告警"] -> w349
              frame Default {
                n202 = Format Into String(format string="%d" ("格式字符串"), initial string="未知" ("工作状态"), w356) -> (resulting string=w355:string)  [unwired: 1 in, 1 out]
              }
              frame "无告警" {
              }
              frame "缺试剂告警" {
              }
              frame "缺水样告警" {
              }
              frame "缺蒸馏水告警" {
              }
              frame "缺标液告警" {
              }
              frame "仪表漏液告警" {
              }
              frame "标定异常告警" {
              }
              frame "超量程告警" {
              }
              frame "加热异常" {
              }
              frame "低试剂预警" {
              }
              frame "超上限告警" {
              }
              frame "超下限告警" {
              }
              frame "仪表内部其他异常" {
              }
              frame "滴定异常告警" {
              }
              frame "电极异常告警" {
              }
              frame "量程切换告警" {
              }
              frame "参数设置告警" {
              }
              frame "PH电极电位异常" {
              }
              frame "电导率电极异常" {
              }
              frame "浊度光度异常" {
              }
              frame "溶解氧电极异常" {
              }
              frame "溶解氧光强异常" {
              }
              frame "温度异常告警" {
              }
              frame "PH异常告警" {
              }
              frame "溶解氧异常告警" {
              }
              frame "电导率异常告警" {
              }
              frame "浊度异常告警" {
              }
              frame "叶绿素异常告警" {
              }
              frame "藻密度异常告警" {
              }
              frame "蓝绿藻异常告警" {
              }
              frame "ORP异常告警" {
              }
              frame "氨氮异常告警" {
              }
              frame "清洁刷异常告警" {
              }
              frame "SD卡异常告警" {
              }
              frame "蓝牙异常告警" {
              }
              frame "Wifi异常告警" {
              }
              frame "流程异常告警" {
              }
            }
            n203 = case shown="3, 92" w354 {
              tunnel: ["总磷" ("table输入") "氨氮" ("table输入") "总氮" ("table输入")] -> w350
              frame 1, 131 {
              }
              frame 3, 92 {
              }
              frame 2, 76, Default {
              }
            }
            n204 = Get Date/Time In Seconds() -> (seconds since 1Jan1904=w351:timestamp)
            n205 = Bundle By Name(cluster=T17 {"时间标识"=timestamp(0 s since 1904-01-01), "设备"="", "日志信息"=""} ("data in"), "时间标识"=w351, "设备"=w350, "日志信息"=w349) -> (w352:T17)
            n206 = call "氨氮报警信息.vi"("data in"=w352) -> ()  [unwired: 10 in, 1 out]
          }
        }
      }
    }
  }
  n207 = while {
    tunnel: w10 -> [w432]
    tunnel: [w430] -> _
    stop <- FALSE stop-if-true
    # "定时更新"
    n208 = Get Queue Status(queue=w432) -> (queue out=w429:refnum<queue>, # elements in queue=w428:i32)  [unwired: 2 in, 6 out]
    n209 = case shown="0" w428 {
      tunnel: [_ w435] -> w430
      tunnel: w429 -> [_ w434]
      frame Default {
      }
      frame 0 {
        w438 = u16 3 items=["总磷"=1, "氨氮"=3] ("站号")
        n210 = call "版本号读取.vi"() -> ("error out"=w435:errorcluster, "固件版本号"=→"固件版本号":string)  [unwired: 10 in]
        n211 = Bundle By Name(cluster=cluster{"命令":string, "data":variant} {"命令"="", "data"=variant} ("元素"), "命令"="读序列号", "data"=w438) -> (w437:cluster{"命令":string, "data":variant})
        n212 = Enqueue Element(queue=w434, element=w437) -> ()  [unwired: 2 in, 3 out]
      }
    }
    n213 = Wait (ms)(milliseconds to wait=u32 1000 ("等待时间（毫秒）")) -> ()  [unwired: 1 out]
  }
  n214 = property on="曲线模型" class="曲线模型 (严格)"("属性"=w1) -> (error out=w9:errorcluster)  [unwired: 2 in, 1 out]
  n215 = Cancel Notification(0:w6) -> (8:w5:refnum<notifier>)  [unwired: 1 in, 2 out]
  n216 = Obtain Queue(name (unnamed)="NH3N" ("名称（未命名）"), element data type=cluster{"命令":string, "data":variant} {"命令"="", "data"=variant}) -> (queue out=w20:refnum<queue>, error out=w21:errorcluster)  [unwired: 3 in, 1 out]
  n217 = while {
    tunnel: w20 -> [w446]
    tunnel: w21 -> [_]
    stop <- FALSE stop-if-true
    n218 = Get Queue Status(queue=w446) -> (queue out=w442:refnum<queue>, # elements in queue=w441:i32)  [unwired: 2 in, 6 out]
    n219 = Wait (ms)(milliseconds to wait=u32 1000 ("等待时间（毫秒）")) -> ()  [unwired: 1 out]
    n220 = global read "氨氮断电保存全局变量.vi" "流程路径"() -> (w445:path)
    n221 = case shown="0" w441 {
      tunnel: w442 -> [_ w449]
      frame Default {
      }
      frame 0 {
        w458 = u16 3 items=["总磷"=1, "氨氮"=3] ("站号")
        # "试剂填充 172 \n管路清洗108\n氨氮92\n总磷131\n总磷海水147\n总氮76\n总氮海水92"
        n222 = global read "VAR氨氮全局变量.vi" "状态告警区"() -> (w450:T4)
        n223 = Bundle By Name(cluster=cluster{"命令":string, "data":variant} {"命令"="", "data"=variant} ("元素"), "命令"="读状态告警区", "data"=w458) -> (w464:cluster{"命令":string, "data":variant})
        n224 = Bundle By Name(cluster=cluster{"命令":string, "data":variant} {"命令"="", "data"=variant} ("元素"), "命令"="读测量数据区", "data"=w458) -> (w461:cluster{"命令":string, "data":variant})
        n225 = Unbundle By Name(w450) -> ("系统时间"=w457:timestamp)
        n226 = Enqueue Element(queue=w449, element=w464) -> (queue out=w459:refnum<queue>)  [unwired: 2 in, 2 out]
        n227 = Get Date/Time In Seconds() -> (seconds since 1Jan1904=w456:timestamp)
        n228 = Subtract(x=w456, y=w457) -> (x-y=w455:dbl)
        n229 = Absolute Value(x=w455) -> (abs(x)=w454:dbl)
        n230 = Enqueue Element(queue=w459, element=w461) -> (queue out=w451:refnum<queue>)  [unwired: 2 in, 2 out]
        n231 = Greater Or Equal?(x=w454, y=120.0) -> (x >= y?=w452:bool)
        n232 = case shown="真" w452 {
          tunnel: w451 -> [_ w467]
          frame False {
          }
          frame True {
            n233 = call "氨氮启动命令.vi"("参数"=T20 {"站号"=3, "量程切换"=enum."AUTO", "控制命令"=enum."校时", "模式设置"=enum."待机", "测量间隔"=0}) -> ("启动命令"=w466:cluster{"命令":string, "data":variant})  [unwired: 10 in]
            n234 = Enqueue Element(queue=w467, element=w466) -> ()  [unwired: 2 in, 3 out]
          }
        }
      }
    }
    n235 = local write "流程路径"(w445) -> ()
    n236 = global read "氨氮断电保存全局变量.vi" "MB通信方式选择"() -> (w443:enum16{"串口", "TCP"})
    n237 = case shown="\"TCP\"" w443 {
      tunnel: [w469 w470] -> w444
      frame "串口", Default {
        n238 = global read "氨氮断电保存全局变量.vi" "VISA Resource"() -> (w469:refnum<visa-resource-name>)
      }
      frame "TCP" {
        n239 = global read "氨氮断电保存全局变量.vi" "IP"() -> (w470:string)
      }
    }
    "字符串" <- w444
  }
  n240 = control-ref of="测量模式下拉列表"() -> (w17:refnum<vi>)
  n241 = control-ref of="量程切换阈值"() -> (w15:refnum<vi>)
  n242 = control-ref of="参数下拉列表"() -> (w18:refnum<vi>)
  n243 = control-ref of="量程下拉列表"() -> (w19:refnum<vi>)
  n244 = control-ref of="备用系数"() -> (w14:refnum<vi>)
  n245 = control-ref of="公式"() -> (w16:refnum<vi>)
  n246 = while {
    tunnel: w20 -> [w478]
    tunnel: w19 -> [w477]
    tunnel: w18 -> [w476]
    tunnel: w17 -> [w475]
    tunnel: w16 -> [w474]
    tunnel: w15 -> [w473]
    tunnel: w14 -> [w472]
    tunnel: w9 -> [_]
    tunnel: w5 -> [w471]
    stop <- FALSE stop-if-true
    n247 = event shown="[14] \"停止\": 值改变" {
      selector: _ -> [_ _ _ _ _ _ _ _ _ _ _ _ _ _ _ _ _ _ _ _ _ _ _ _]
      dyn-events: _ -> [_ _ _ _ _ _ _ _ _ _ _ _ _ _ _ _ _ _ _ _ _ _ _ _]
      timeout: _ -> [_ _ _ _ _ _ _ _ _ _ _ _ _ _ _ _ _ _ _ _ _ _ _ _]
      tunnel: w478 -> [_ _ w494 w522 _ _ _ _ _ _ _ w625 _ w650 w657 _ _ _ _ _ _ _ _ _]
      tunnel: w477 -> [_ _ _ _ _ _ _ _ _ _ _ _ _ _ _ _ _ _ w673 _ w693 w702 w708 w720]
      tunnel: w476 -> [_ _ _ _ _ _ _ _ _ _ _ _ _ _ _ _ _ _ w671 _ w691 w704 w716 w727]
      tunnel: w475 -> [_ _ _ _ _ _ _ _ _ _ _ _ _ _ _ _ _ _ w672 _ w692 w703 w710 w722]
      tunnel: w474 -> [_ _ _ _ _ _ _ _ _ _ _ _ _ _ _ _ _ _ w667 _ _ _ _ _]
      tunnel: w473 -> [_ _ _ _ _ _ _ _ _ _ _ _ _ _ _ _ _ _ _ _ w687 _ _ _]
      tunnel: w472 -> [_ _ _ _ _ _ _ _ _ _ _ _ _ _ _ _ _ _ _ _ _ _ w714 _]
      tunnel: w471 -> [_ _ _ _ _ _ _ _ _ _ _ _ _ _ w653 _ _ _ _ _ _ _ _ _]
      tunnel: [_ w480 _ _ _ _ _ _ _ _ _ _ _ _ _ _ _ _ _ _ _ _ _ _] -> _
      event Timeout {
        n248 = event-data() -> ()  [unwired: 1 in, 3 out]
      }
      event "测量模式下拉列表", "量程下拉列表", "参数下拉列表": Value Change {
        n249 = event-data() -> ()  [unwired: 1 in, 6 out]
        n250 = local read "参数下拉列表"() -> (w481:enum16{"总磷", "总氮", "氨氮"})
        n251 = local read "测量模式下拉列表"() -> (w482:enum16{"水样测量", "零点核查", "跨度核查", "标样核查", "加标回收"})
        n252 = local read "量程下拉列表"() -> (w483:enum16{"低量程", "高量程"})
        n253 = Bundle("参数下拉列表"=w481, "测量模式下拉列表"=w482, "量程下拉列表"=w483) -> (w484:T14)  [unwired: 1 in]
        n254 = property on="曲线模型" class="曲线模型 (严格)"("属性"=w484) -> (error out=w480:errorcluster)  [unwired: 2 in, 1 out]
      }
      event "串口设置": Value Change {
        n255 = event-data() -> ()  [unwired: 1 in, 6 out]
        n256 = global read "氨氮断电保存全局变量.vi" "MB通信方式选择"() -> (w485:enum16{"串口", "TCP"})
        n257 = global read "氨氮断电保存全局变量.vi" "VISA Resource"() -> (w491:refnum<visa-resource-name>)
        n258 = global read "氨氮断电保存全局变量.vi" "PORT"() -> (w489:string)
        n259 = global read "氨氮断电保存全局变量.vi" "IP"() -> (w490:string)
        n260 = call "串口配置.vi"("PORT"=w489, "IP"=w490, "MB通信方式选择"=w485, "请选择串口:"=w491) -> ("PORT 2"=w487:string, "IP 2"=w488:string, "确认 2"=w492:bool, "VISA资源名称 2"=w493:refnum<visa-resource-name>, "MB通信方式选择 2"=w486:enum16{"串口", "TCP"})  [unwired: 3 in]
        n261 = case shown="真" w492 {
          tunnel: w493 -> [_ w499]
          tunnel: w494 -> [_ w498]
          tunnel: w488 -> [_ w497]
          tunnel: w487 -> [_ w496]
          tunnel: w486 -> [_ w495]
          frame False {
          }
          frame True {
            n262 = flat-sequence {
              tunnel: w499 -> [w504]
              tunnel: w498 -> [w505]
              tunnel: w497 -> [w503]
              tunnel: w496 -> [w502]
              tunnel: w495 -> [w501]
              frame #0 {
                n263 = global write "氨氮断电保存全局变量.vi" "IP"(w503) -> ()
                n264 = global write "氨氮断电保存全局变量.vi" "PORT"(w502) -> ()
                n265 = global write "氨氮断电保存全局变量.vi" "VISA Resource"(w504) -> ()
                n266 = global write "氨氮断电保存全局变量.vi" "MB通信方式选择"(w501) -> ()
                n267 = Flush Queue(queue=w505) -> (queue out=w500:refnum<queue>)  [unwired: 1 in, 2 out]
                n268 = Enqueue Element(queue=w500, element=cluster{"命令":string, "data":variant} {"命令"="启用模块", "data"=variant} ("元素")) -> ()  [unwired: 2 in, 3 out]
              }
              frame #1 {
                n269 = call <vilib>:"Application Directory.vi"() -> ("Application Directory"=w520:path)
                n270 = Build Path(base path=w520, name or relative path="data\\sys.ini" ("名称或相对路径")) -> (appended path=w518:path)
                n271 = call <vilib>:"Open Config Data.vi"("configuration file path"=w518) -> ("error out"=w514:errorcluster, "refnum"=w517:T13)  [unwired: 8 in, 1 out]
                n272 = vi-ref "氨氮断电保存全局变量.vi"() -> (w516:refnum<vi>)
                n273 = call <userlib>:"Write Panel to INI__ogtk.vi"("error in (no error)"=w514, "VI ref"=w516, "refnum"=w517) -> ("error out"=w513:errorcluster, "refnum out"=w515:T13)  [unwired: 7 in]
                n274 = call <vilib>:"Close Config Data.vi"("error in (no error)"=w513, "refnum"=w515) -> ("error out"=w508:errorcluster, "file path"=w507:path)  [unwired: 8 in]
                n275 = Open/Create/Replace File(file path (use dialog)=w507, error in=w508) -> (refnum out=w511:refnum<file>, error out=w512:errorcluster)  [unwired: 4 in, 1 out]
                n276 = Flush File(refnum=w511, error in=w512) -> (refnum out=w510:refnum<file>, error out=w509:errorcluster)
                n277 = Close File(refnum=w510, error in=w509) -> ()  [unwired: 2 out]
              }
            }
          }
        }
      }
      event "模块启用": Value Change {
        n278 = event-data() -> ("OldVal"=w523:bool)  [unwired: 1 in, 5 out]
        n279 = Flush Queue(queue=w522) -> (queue out=w521:refnum<queue>)  [unwired: 1 in, 2 out]
        n280 = case shown="假" w523 {
          tunnel: w521 -> [w524 w526]
          frame False {
            n281 = Enqueue Element(queue=w524, element=cluster{"命令":string, "data":variant} {"命令"="停用模块", "data"=variant} ("元素")) -> ()  [unwired: 2 in, 3 out]
          }
          frame True {
            n282 = Enqueue Element(queue=w526, element=cluster{"命令":string, "data":variant} {"命令"="启用模块", "data"=variant} ("元素")) -> ()  [unwired: 2 in, 3 out]
          }
        }
      }
      event "流程路径": Value Change {
        n283 = event-data() -> ()  [unwired: 1 in, 6 out]
        n284 = flat-sequence {
          frame #0 {
            n285 = local read "流程路径"() -> (w528:path)
            n286 = global write "氨氮断电保存全局变量.vi" "流程路径"(w528) -> ()
          }
          frame #1 {
            n287 = call <vilib>:"Application Directory.vi"() -> ("Application Directory"=w542:path)
            n288 = Build Path(base path=w542, name or relative path="data\\sys.ini" ("名称或相对路径")) -> (appended path=w540:path)
            n289 = call <vilib>:"Open Config Data.vi"("configuration file path"=w540) -> ("error out"=w536:errorcluster, "refnum"=w539:T13)  [unwired: 8 in, 1 out]
            n290 = vi-ref "氨氮断电保存全局变量.vi"() -> (w538:refnum<vi>)
            n291 = call <userlib>:"Write Panel to INI__ogtk.vi"("error in (no error)"=w536, "VI ref"=w538, "refnum"=w539) -> ("error out"=w535:errorcluster, "refnum out"=w537:T13)  [unwired: 7 in]
            n292 = call <vilib>:"Close Config Data.vi"("error in (no error)"=w535, "refnum"=w537) -> ("error out"=w530:errorcluster, "file path"=w529:path)  [unwired: 8 in]
            n293 = Open/Create/Replace File(file path (use dialog)=w529, error in=w530) -> (refnum out=w533:refnum<file>, error out=w534:errorcluster)  [unwired: 4 in, 1 out]
            n294 = Flush File(refnum=w533, error in=w534) -> (refnum out=w532:refnum<file>, error out=w531:errorcluster)
            n295 = Close File(refnum=w532, error in=w531) -> ()  [unwired: 2 out]
          }
        }
      }
      event "公式一键写入": Value Change {
        n296 = event-data() -> ()  [unwired: 1 in, 6 out]
        n297 = local read "公式"() -> (w543:cluster{"X^2":dbl, "X":dbl, "b":dbl})
        n298 = call "公式复合写入.vi"("公式"=w543) -> ()  [unwired: 11 in]
      }
      event "备用系数一键写入": Value Change {
        n299 = event-data() -> ()  [unwired: 1 in, 6 out]
        n300 = local read "备用系数"() -> (w544:T2)
        n301 = call "量程参数复合参数写入.vi"("备用系数"=w544) -> ()  [unwired: 11 in]
      }
      event "曲线模型": Value Change {
        n302 = event-data() -> ()  [unwired: 1 in, 6 out]
        n303 = local write "公式"("曲线模型") -> ()
      }
      event "质控参数设置": Value Change {
        n304 = event-data() -> ()  [unwired: 1 in, 6 out]
        n305 = global read "氨氮断电保存全局变量.vi" "质控参数设置"() -> (w546:T21)
        n306 = call "氨氮质控参数设置.vi"("质控参数设置"=w546) -> ("输出簇"=w547:T22)  [unwired: 10 in]
        n307 = Unbundle By Name(w547) -> ("确定"=w548:bool)
        n308 = case shown="真" w548 {
          tunnel: w547 -> [_ w550]
          tunnel: w546 -> [_ w549]
          frame False {
          }
          frame True {
            n309 = flat-sequence {
              tunnel: w550 -> [w557]
              tunnel: w549 -> [w556]
              frame #0 {
                n310 = Unbundle By Name(w557) -> ("跨度值"=w555:dbl, "零点标准液浓度"=w554:dbl, "跨度标准液浓度"=w553:dbl, "标准液标准浓度"=w552:dbl)
                n311 = Bundle By Name(cluster=w556, "氨氮跨度值"=w555, "氨氮零点标准液浓度"=w554, "氨氮跨度标准液浓度"=w553, "氨氮标准液标准浓度"=w552) -> (w551:T21)
                n312 = global write "氨氮断电保存全局变量.vi" "质控参数设置"(w551) -> ()
              }
              frame #1 {
                n313 = call <vilib>:"Application Directory.vi"() -> ("Application Directory"=w571:path)
                n314 = Build Path(base path=w571, name or relative path="data\\sys.ini" ("名称或相对路径")) -> (appended path=w569:path)
                n315 = call <vilib>:"Open Config Data.vi"("configuration file path"=w569) -> ("error out"=w565:errorcluster, "refnum"=w568:T13)  [unwired: 8 in, 1 out]
                n316 = vi-ref "氨氮断电保存全局变量.vi"() -> (w567:refnum<vi>)
                n317 = call <userlib>:"Write Panel to INI__ogtk.vi"("error in (no error)"=w565, "VI ref"=w567, "refnum"=w568) -> ("error out"=w564:errorcluster, "refnum out"=w566:T13)  [unwired: 7 in]
                n318 = call <vilib>:"Close Config Data.vi"("error in (no error)"=w564, "refnum"=w566) -> ("error out"=w559:errorcluster, "file path"=w558:path)  [unwired: 8 in]
                n319 = Open/Create/Replace File(file path (use dialog)=w558, error in=w559) -> (refnum out=w562:refnum<file>, error out=w563:errorcluster)  [unwired: 4 in, 1 out]
                n320 = Flush File(refnum=w562, error in=w563) -> (refnum out=w561:refnum<file>, error out=w560:errorcluster)
                n321 = Close File(refnum=w561, error in=w560) -> ()  [unwired: 2 out]
              }
            }
          }
        }
      }
      event "仪器参数设置": Value Change {
        n322 = event-data() -> ()  [unwired: 1 in, 6 out]
        n323 = global read "氨氮断电保存全局变量.vi" "氨氮仪器参数"() -> (w573:T23)
        n324 = call "仪器参数设置.vi"("仪器参数设置"=w573) -> ("仪器参数设置输出"=w572:T24)  [unwired: 10 in]
        n325 = Unbundle By Name(w572) -> ("确定"=w574:bool)
        n326 = case shown="真" w574 {
          tunnel: w572 -> [_ w576]
          tunnel: w573 -> [_ w575]
          frame False {
          }
          frame True {
            n327 = flat-sequence {
              tunnel: w576 -> [w593]
              tunnel: w575 -> [w592]
              frame #0 {
                n328 = Unbundle By Name(w593) -> ("测量量程"=w591:dbl, "测量精度"=w590:dbl, "测量间隔"=w589:dbl, "消解温度"=w588:dbl, "消解时长"=w586:dbl, "空白校准时间"=w585:timestamp, "曲线截距"=w584:dbl, "曲线斜率"=w583:dbl, "测量检出限"=w582:dbl, "测量信号值"=w581:dbl, "线性相关系数"=w580:dbl, "二次多项式系数"=w579:dbl, "标样校准时间"=w578:timestamp, "单位"=w577:u16)
                n329 = Bundle By Name(cluster=w592, "测量量程"=w591, "测量精度"=w590, "测量间隔"=w589, "消解温度"=w588, "消解时长"=w586, "空白校准时间"=w585, "曲线截距"=w584, "曲线斜率"=w583, "测量检出限"=w582, "测量信号值"=w581, "线性相关系数"=w580, "二次多项式系数"=w579, "标样校准时间"=w578, "单位"=w577) -> (w587:T23)
                n330 = global write "氨氮断电保存全局变量.vi" "氨氮仪器参数"(w587) -> ()
              }
              frame #1 {
                n331 = call <vilib>:"Application Directory.vi"() -> ("Application Directory"=w607:path)
                n332 = Build Path(base path=w607, name or relative path="data\\sys.ini" ("名称或相对路径")) -> (appended path=w605:path)
                n333 = call <vilib>:"Open Config Data.vi"("configuration file path"=w605) -> ("error out"=w601:errorcluster, "refnum"=w604:T13)  [unwired: 8 in, 1 out]
                n334 = vi-ref "氨氮断电保存全局变量.vi"() -> (w603:refnum<vi>)
                n335 = call <userlib>:"Write Panel to INI__ogtk.vi"("error in (no error)"=w601, "VI ref"=w603, "refnum"=w604) -> ("error out"=w600:errorcluster, "refnum out"=w602:T13)  [unwired: 7 in]
                n336 = call <vilib>:"Close Config Data.vi"("error in (no error)"=w600, "refnum"=w602) -> ("error out"=w595:errorcluster, "file path"=w594:path)  [unwired: 8 in]
                n337 = Open/Create/Replace File(file path (use dialog)=w594, error in=w595) -> (refnum out=w598:refnum<file>, error out=w599:errorcluster)  [unwired: 4 in, 1 out]
                n338 = Flush File(refnum=w598, error in=w599) -> (refnum out=w597:refnum<file>, error out=w596:errorcluster)
                n339 = Close File(refnum=w597, error in=w596) -> ()  [unwired: 2 out]
              }
            }
          }
        }
      }
      event "自动测试量程配置": Value Change {
        n340 = event-data() -> ()  [unwired: 1 in, 6 out]
        n341 = flat-sequence {
          frame #0 {
            n342 = global write "氨氮断电保存全局变量.vi" "氨氮自动测试量程配置"("自动测试量程配置") -> ()
          }
          frame #1 {
            n343 = call <vilib>:"Application Directory.vi"() -> ("Application Directory"=w622:path)
            n344 = Build Path(base path=w622, name or relative path="data\\sys.ini" ("名称或相对路径")) -> (appended path=w620:path)
            n345 = call <vilib>:"Open Config Data.vi"("configuration file path"=w620) -> ("error out"=w616:errorcluster, "refnum"=w619:T13)  [unwired: 8 in, 1 out]
            n346 = vi-ref "氨氮断电保存全局变量.vi"() -> (w618:refnum<vi>)
            n347 = call <userlib>:"Write Panel to INI__ogtk.vi"("error in (no error)"=w616, "VI ref"=w618, "refnum"=w619) -> ("error out"=w615:errorcluster, "refnum out"=w617:T13)  [unwired: 7 in]
            n348 = call <vilib>:"Close Config Data.vi"("error in (no error)"=w615, "refnum"=w617) -> ("error out"=w610:errorcluster, "file path"=w609:path)  [unwired: 8 in]
            n349 = Open/Create/Replace File(file path (use dialog)=w609, error in=w610) -> (refnum out=w613:refnum<file>, error out=w614:errorcluster)  [unwired: 4 in, 1 out]
            n350 = Flush File(refnum=w613, error in=w614) -> (refnum out=w612:refnum<file>, error out=w611:errorcluster)
            n351 = Close File(refnum=w612, error in=w611) -> ()  [unwired: 2 out]
          }
        }
      }
      event "手动启动": Value Change {
        n352 = event-data() -> ()  [unwired: 1 in, 6 out]
        n353 = call "氨氮启动参数对话框.vi"() -> ("确认"=w623:bool, "元素"=w624:cluster{"命令":string, "data":variant})  [unwired: 10 in]
        n354 = case shown="真" w623 {
          tunnel: w625 -> [_ w627]
          tunnel: w624 -> [_ w626]
          frame False {
          }
          frame True {
            n355 = Enqueue Element(queue=w627, element=w626) -> ()  [unwired: 2 in, 3 out]
          }
        }
      }
      event "定时启动": Mouse Down {
        n356 = event-data() -> ()  [unwired: 1 in, 6 out]
        n357 = flat-sequence {
          frame #0 {
            n358 = global read "氨氮断电保存全局变量.vi" "定时控制"() -> (w629:T6)
            n359 = call "周期设置.vi"("定时控制输入"=w629) -> ("定时控制输出"=w628:T25)  [unwired: 10 in]
            n360 = global write "氨氮断电保存全局变量.vi" "定时控制"(w628) -> ()
          }
          frame #1 {
            n361 = call <vilib>:"Application Directory.vi"() -> ("Application Directory"=w643:path)
            n362 = Build Path(base path=w643, name or relative path="data\\sys.ini" ("名称或相对路径")) -> (appended path=w641:path)
            n363 = call <vilib>:"Open Config Data.vi"("configuration file path"=w641) -> ("error out"=w637:errorcluster, "refnum"=w640:T13)  [unwired: 8 in, 1 out]
            n364 = vi-ref "氨氮断电保存全局变量.vi"() -> (w639:refnum<vi>)
            n365 = call <userlib>:"Write Panel to INI__ogtk.vi"("error in (no error)"=w637, "VI ref"=w639, "refnum"=w640) -> ("error out"=w636:errorcluster, "refnum out"=w638:T13)  [unwired: 7 in]
            n366 = call <vilib>:"Close Config Data.vi"("error in (no error)"=w636, "refnum"=w638) -> ("error out"=w631:errorcluster, "file path"=w630:path)  [unwired: 8 in]
            n367 = Open/Create/Replace File(file path (use dialog)=w630, error in=w631) -> (refnum out=w634:refnum<file>, error out=w635:errorcluster)  [unwired: 4 in, 1 out]
            n368 = Flush File(refnum=w634, error in=w635) -> (refnum out=w633:refnum<file>, error out=w632:errorcluster)
            n369 = Close File(refnum=w633, error in=w632) -> ()  [unwired: 2 out]
          }
        }
      }
      event "单步测试": Value Change {
        w645 = u16 1 items=["总磷"=1, "氨氮"=3] ("站号")
        n370 = event-data() -> ()  [unwired: 1 in, 6 out]
        n371 = Bundle("站号"=w645, "总磷氨氮调试"="总磷氨氮调试") -> (w644:cluster{"站号":u16, "总磷氨氮调试":u16[]})  [unwired: 1 in]
        n372 = Bundle By Name(cluster=cluster{"命令":string, "data":variant} {"命令"="", "data"=variant} ("元素"), "命令"="debug", "data"=w644) -> (w647:cluster{"命令":string, "data":variant})
        n373 = Enqueue Element(queue=w650, element=w647) -> ()  [unwired: 2 in, 3 out]
      }
      event "停止": Value Change {
        n374 = event-data() -> ()  [unwired: 1 in, 6 out]
        n375 = Enqueue Element(queue=w657, element=cluster{"命令":string, "data":variant} {"命令"="启动", "data"=variant(cluster{"站号":u16, "控制命令输出":u16[]} {"站号"=1, "控制命令输出"=[2816]})} ("元素")) -> (queue out=w655:refnum<queue>)  [unwired: 2 in, 2 out]
        n376 = Cancel Notification(0:w653) -> (8:w654:refnum<notifier>)  [unwired: 1 in, 2 out]
        n377 = Send Notification(notification=TRUE ("通知"), notifier=w654) -> ()  [unwired: 1 in, 2 out]
        n378 = Enqueue Element(queue=w655, element=cluster{"命令":string, "data":variant} {"命令"="启动", "data"=variant(cluster{"站号":u16, "控制命令":u16[]} {"站号"=3, "控制命令"=[2816]})} ("启动命令")) -> ()  [unwired: 2 in, 3 out]
      }
      event "设置": Value Change {
        n379 = event-data() -> ()  [unwired: 1 in, 6 out]
        n380 = property on="窗格" class="Pane"("Origin"=T11 {"Horizontal"=0, "Vertical"=628} ("原点")) -> ()  [unwired: 2 in, 2 out]
      }
      event "返回": Value Change {
        n381 = event-data() -> ()  [unwired: 1 in, 6 out]
        n382 = property on="窗格" class="Pane"("Origin"=T11 {"Horizontal"=0, "Vertical"=0} ("原点")) -> ()  [unwired: 2 in, 2 out]
      }
      event "公式.X^2", "公式.X", "公式.b", "量程切换阈值.阈值", "量程切换阈值.标液浓度", "备用系数.量程上限", "备用系数.量程下限", "备用系数.检出限", "备用系数.精度": Mouse Down {
        n383 = event-data() -> ("CtlRef"=w663:refnum<vi>)  [unwired: 1 in, 5 out]
        n384 = property class="DigNum (严格)"(reference=w663) -> (reference out=w661:refnum<vi>, "Value"=w662:dbl)  [unwired: 1 in, 1 out]
        n385 = call "数字键盘.vi"("OldNumber"=w662) -> ("NewNumber"=w660:dbl)
        n386 = property class="DigNum (严格)"(reference=w661, "Val(Sgnl)"=w660) -> ()  [unwired: 1 in, 2 out]
      }
      event "读公式": Value Change {
        n387 = event-data() -> ()  [unwired: 1 in, 6 out]
        n388 = property class="Enum (严格)"(reference=w671) -> ("Value"=w670:enum16{"总磷", "总氮", "氨氮"})  [unwired: 1 in, 2 out]
        n389 = property class="Enum (严格)"(reference=w672) -> ("Value"=w669:enum16{"水样测量", "零点核查", "跨度核查", "标样核查", "加标回收"})  [unwired: 1 in, 2 out]
        n390 = property class="Enum (严格)"(reference=w673) -> ("Value"=w668:enum16{"低量程", "高量程"})  [unwired: 1 in, 2 out]
        n391 = call "公式读取.vi"("量程"=w668, "测量模式"=w669, "测量参数"=w670) -> ("error out"=w665:errorcluster, "公式"=w666:cluster{"X^2":dbl, "X":dbl, "b":dbl})  [unwired: 7 in]
        n392 = property class="Clust (严格)"(reference=w667, "Value"=w666) -> ()  [unwired: 1 in, 2 out]
        n393 = case shown="错误" w665 {
          tunnel: ["读取成功" ("消息") "读取失败" ("消息")] -> w664
          frame No Error {
          }
          frame Error {
          }
        }
        n394 = One Button Dialog(message=w664) -> ()  [unwired: 1 in, 1 out]
      }
      event "写公式": Value Change {
        n395 = event-data() -> ()  [unwired: 1 in, 6 out]
        n396 = call "公式写入.vi"("公式"="公式", "量程"="量程下拉列表", "测量模式"="测量模式下拉列表", "测量参数"="参数下拉列表") -> ("error out"=w678:errorcluster)  [unwired: 7 in]
        n397 = case shown="无错误" w678 {
          tunnel: ["写入成功" ("消息") "写入失败" ("消息")] -> w679
          frame No Error {
          }
          frame Error {
          }
        }
        n398 = One Button Dialog(message=w679) -> ()  [unwired: 1 in, 1 out]
      }
      event "量程切换阈值读取": Value Change {
        n399 = event-data() -> ()  [unwired: 1 in, 6 out]
        n400 = property class="Enum (严格)"(reference=w691) -> ("Value"=w690:enum16{"总磷", "总氮", "氨氮"})  [unwired: 1 in, 2 out]
        n401 = property class="Enum (严格)"(reference=w692) -> ("Value"=w689:enum16{"水样测量", "零点核查", "跨度核查", "标样核查", "加标回收"})  [unwired: 1 in, 2 out]
        n402 = property class="Enum (严格)"(reference=w693) -> ("Value"=w688:enum16{"低量程", "高量程"})  [unwired: 1 in, 2 out]
        n403 = call "量程读取.vi"("量程"=w688, "测量模式"=w689, "测量参数"=w690) -> ("error out"=w684:errorcluster, "量程切换阈值"=w686:cluster{"阈值":dbl, "标液浓度":dbl})  [unwired: 7 in]
        n404 = property class="Clust (严格)"(reference=w687, "Value"=w686) -> ()  [unwired: 1 in, 2 out]
        n405 = case shown="错误" w684 {
          tunnel: ["读取成功" ("消息") "读取失败" ("消息")] -> w685
          frame No Error {
          }
          frame Error {
          }
        }
        n406 = One Button Dialog(message=w685) -> ()  [unwired: 1 in, 1 out]
      }
      event "量程切换阈值写入": Value Change {
        n407 = event-data() -> ()  [unwired: 1 in, 6 out]
        n408 = property class="Enum (严格)"(reference=w704) -> ("Value"=w701:enum16{"总磷", "总氮", "氨氮"})  [unwired: 1 in, 2 out]
        n409 = property class="Enum (严格)"(reference=w703) -> ("Value"=w700:enum16{"水样测量", "零点核查", "跨度核查", "标样核查", "加标回收"})  [unwired: 1 in, 2 out]
        n410 = property class="Enum (严格)"(reference=w702) -> ("Value"=w699:enum16{"低量程", "高量程"})  [unwired: 1 in, 2 out]
        n411 = call "量程写入.vi"("量程切换阈值"="量程切换阈值", "量程"=w699, "测量模式"=w700, "测量参数"=w701) -> ("error out"=w696:errorcluster)  [unwired: 7 in]
        n412 = case shown="无错误" w696 {
          tunnel: ["写入成功" ("消息") "写入失败" ("消息")] -> w697
          frame No Error {
          }
          frame Error {
          }
        }
        n413 = One Button Dialog(message=w697) -> ()  [unwired: 1 in, 1 out]
      }
      event "备用系数读取": Value Change {
        n414 = event-data() -> ()  [unwired: 1 in, 6 out]
        n415 = property class="Enum (严格)"(reference=w716) -> ("Value"=w715:enum16{"总磷", "总氮", "氨氮"})  [unwired: 1 in, 2 out]
        n416 = property class="Enum (严格)"(reference=w710) -> ("Value"=w709:enum16{"水样测量", "零点核查", "跨度核查", "标样核查", "加标回收"})  [unwired: 1 in, 2 out]
        n417 = property class="Enum (严格)"(reference=w708) -> ("Value"=w707:enum16{"低量程", "高量程"})  [unwired: 1 in, 2 out]
        n418 = call "备用系数读取.vi"("量程"=w707, "测量模式"=w709, "测量参数"=w715) -> ("error out"=w711:errorcluster, "备用系数"=w713:T2)  [unwired: 7 in]
        n419 = property class="Clust (严格)"(reference=w714, "Value"=w713) -> ()  [unwired: 1 in, 2 out]
        n420 = case shown="错误" w711 {
          tunnel: ["读取成功" ("消息") "读取失败" ("消息")] -> w712
          frame No Error {
          }
          frame Error {
          }
        }
        n421 = One Button Dialog(message=w712) -> ()  [unwired: 1 in, 1 out]
      }
      event "备用系数写入": Value Change {
        n422 = event-data() -> ()  [unwired: 1 in, 6 out]
        n423 = property class="Enum (严格)"(reference=w727) -> ("Value"=w726:enum16{"总磷", "总氮", "氨氮"})  [unwired: 1 in, 2 out]
        n424 = property class="Enum (严格)"(reference=w722) -> ("Value"=w721:enum16{"水样测量", "零点核查", "跨度核查", "标样核查", "加标回收"})  [unwired: 1 in, 2 out]
        n425 = property class="Enum (严格)"(reference=w720) -> ("Value"=w719:enum16{"低量程", "高量程"})  [unwired: 1 in, 2 out]
        n426 = call "备用系数写入.vi"("备用系数"="备用系数", "量程"=w719, "测量模式"=w721, "测量参数"=w726) -> ("error out"=w723:errorcluster)  [unwired: 7 in]
        n427 = case shown="无错误" w723 {
          tunnel: ["写入成功" ("消息") "写入失败" ("消息")] -> w724
          frame No Error {
          }
          frame Error {
          }
        }
        n428 = One Button Dialog(message=w724) -> ()  [unwired: 1 in, 1 out]
      }
    }
  }
